vi "Init.vi"(8 "error in (no error)":errorcluster, 10 "JQMHStartup.lvclass":refnum<class "JQMHStartup.lvclass">, 11 "JQMHCore.lvclass":refnum<class "JQMHModule.lvclass">) -> (0 "error out":errorcluster, 1 "StartupParams":variant, 3 "JQMHCore out":refnum<class "JQMHModule.lvclass">)   [LabVIEW 2024, in "JQMHShared.lvlib"]
uses:
  JQMHShared.lvlib
  JQMHStartup/JQMHStartup.lvclass
  Module/JQMHModule.lvclass
  JQMHStartup/JQMHStartup.lvclass/JQMHStartup.ctl
  Watchdog/Watchdog.lvclass
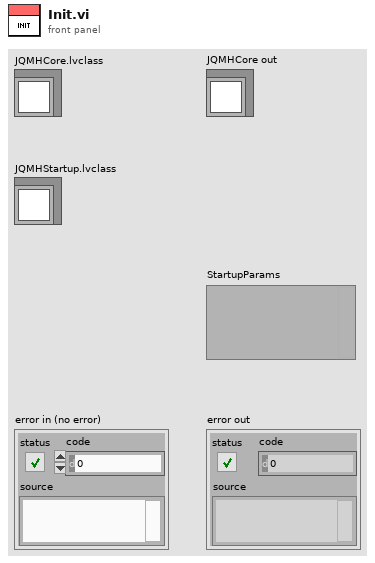
[diagram p1: front panel]
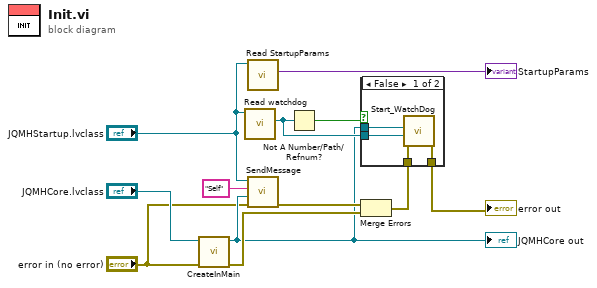
[diagram p0: block diagram]
diagram:
  n1 = call "CreateInMain.vi"("error in (no error)"="error in (no error)", "JQMHModule in"="JQMHCore.lvclass") -> ("error out"=w10:errorcluster, "JQMHModule out"=w2:refnum<class "JQMHModule.lvclass">)  [unwired: 8 in]
  "JQMHCore out" <- w2
  n2 = call "Read watchdog.vi"("JQMHStartup in"="JQMHStartup.lvclass") -> ("watchdog"=w5:refnum<queue>)  [unwired: 8 in, 2 out]
  n3 = call "Read StartupParams.vi"("JQMHStartup in"="JQMHStartup.lvclass") -> ("StartupParams"=→"StartupParams":variant)  [unwired: 8 in, 2 out]
  n4 = call "SendMessage.vi"("error in (no error)"="error in (no error)", "Data"=w2, "Command"="Self", "JQMHStartup in"="JQMHStartup.lvclass") -> ("error out"=w11:errorcluster)  [unwired: 6 in, 1 out]
  n5 = Not A Number/Path/Refnum?(number/path/refnum=w5) -> (NaN/Path/Refnum?=w6:bool)
  n6 = Merge Errors(w11, w10) -> (w4:errorcluster)
  n7 = case shown="False" w6 {
    tunnel: w2 -> [w16 _]
    tunnel: w5 -> [w15 _]
    tunnel: w4 -> [w14 w17]
    tunnel: [w13 w17] -> w3
    frame False {
      n8 = call "Start_WatchDog.vi"("error in (no error)"=w14, "Caller"=w15, "ModToWatch"=w16) -> ("error out"=w13:errorcluster)  [unwired: 8 in]
    }
    frame True {
    }
  }
  "error out" <- w3
